vi "Init.vi"(8 "error in":errorcluster, 11 "Action Point in":refnum<class "Action Point.lvclass">) -> (0 "error out":errorcluster, 3 "Action Point out":refnum<class "Action Point.lvclass">)   [LabVIEW 2024, in "Action Point.lvclass"]
uses:
  Action Point.lvclass
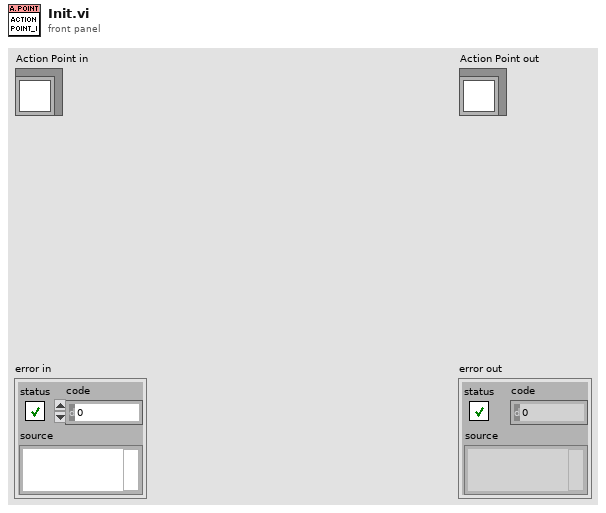
[diagram p1: front panel]
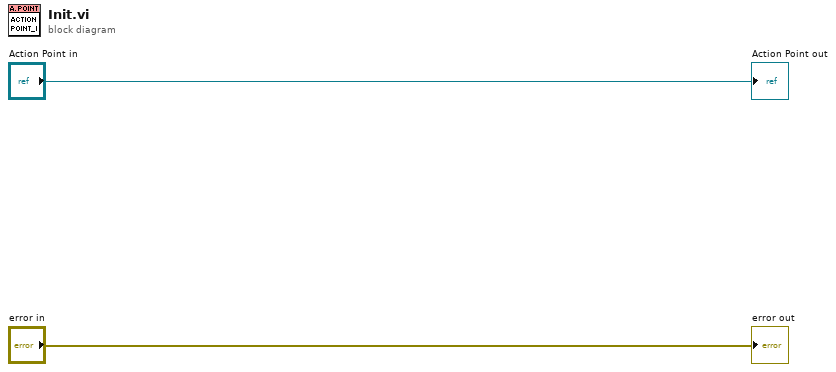
[diagram p0: block diagram]
diagram:
  "error out" <- "error in"
  "Action Point out" <- "Action Point in"
